vi "CVT1ParallelStaticTest.vi"() -> (3 "Unit Test Framework Results":T1)   [LabVIEW 2013, in "UnitTests.lvlib"]
uses:
  UnitTests.lvlib
  <vilib>/utf/common/utf_test_result_troll.ctl
  <vilib>/utf/common/utf_test_result.ctl
  <vilib>/utf/common/utf_test_result_failure.ctl
  <vilib>/utf/common/utf_test_comparison_operators.ctl
  <vilib>/utf/common/utf_vi_tag.ctl
  <vilib>/NI/Current Value Table/Static Write.vi
  <vilib>/NI/Current Value Table/DataTypes/I32_Static Write.vi
  <vilib>/NI/Current Value Table/Static Read.vi
  <vilib>/NI/Current Value Table/DataTypes/I32_Static Read.vi
  <vilib>/NI/Current Value Table/Type to Enum.vi
  <vilib>/NI/Current Value Table/DataTypes/I32_Type To Enum.vi
  <vilib>/NI/Current Value Table/Compatibility/TagConverter.vi
  <vilib>/NI/Current Value Table/Create Tags.vi
  <vilib>/NI/Current Value Table/FGVs/Tag Memory.vi
  <vilib>/NI/Current Value Table/Memory Block.vi
  <vilib>/NI/Current Value Table/DataTypes/I32_Memory Block.vi
  <vilib>/utf/NI_UnitTestFramework.lvlib
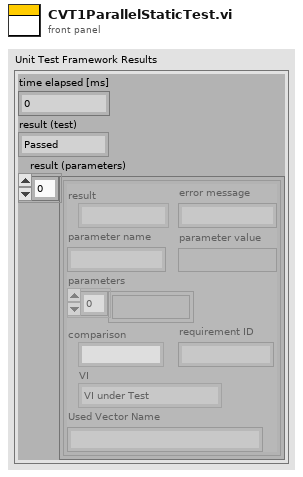
[diagram p1: front panel]
types:
  T1 = typedef "NI_UnitTestFramework.lvlib/utf_test_result_troll.ctl" = cluster{"time elapsed [ms]":u32, "result (test)":T2, "result (parameters)":T3[]}
  T2 = typedef "NI_UnitTestFramework.lvlib/utf_test_result.ctl" = enum16{"Passed", "Failed", "Error", "Skipped", "Not Processed"}
  T3 = typedef "NI_UnitTestFramework.lvlib/utf_test_result_failure.ctl" = cluster{"result":T2, "error message":string, "parameter name":string, "parameter value":variant, "parameters":variant[], "comparison":T4, "requirement ID":string, "VI":T5, "Used Vector Name":string}
  T4 = typedef "NI_UnitTestFramework.lvlib/utf_test_comparison_operators.ctl" = enum16{"=", "!=", ">", ">=", "<", "<=", "range", "symmetric tolerance", "asymmetric tolerance", "string contains", "string not contain", "array size", "string length", "array range", "by element", "array range (limit array)", "user-defined", "array contains", "array not contain", "vector length", "= (elm)", "!= (elm)", "= (case insensitive)", "!= (case insensitive)"}
  T5 = typedef "NI_UnitTestFramework.lvlib/utf_vi_tag.ctl" = enum16{"Setup VI", "VI under Test", "Teardown VI"}
  T6 = typedef "cvt_Tag Configuration.ctl" = cluster{"Name":string, "Data Type":T7, "Array":bool, "Size":u32, "Default":string, "Enum":string[], "Description":string}
  T7 = typedef "cvt_Data Types.ctl" = enum16{"Bool", "U8", "I32", "Double", "String", "Enum"}
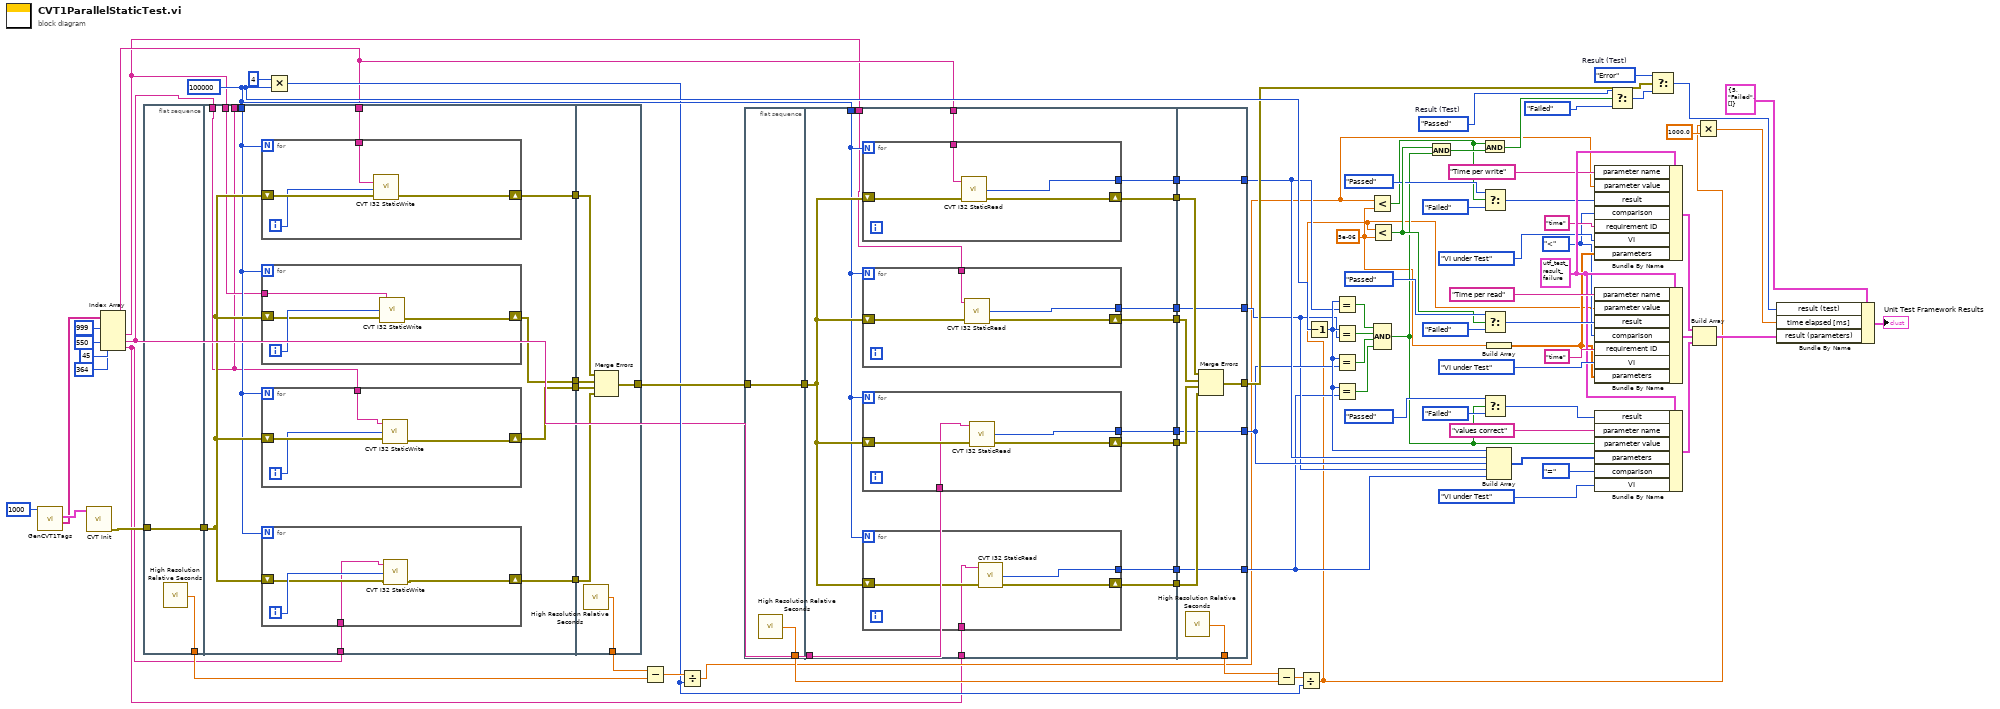
[diagram p0: block diagram]
diagram:
  w38 = T3 {"result"=enum."Passed", "error message"="", "parameter name"="", "parameter value"=variant, "parameters"=[], "comparison"=enum."=", "requirement ID"="", "VI"=enum."Setup VI", "Used Vector Name"=""} ("Unit Test Framework - result (parameters)")
  w18 = 5e-06 ("y")
  w29 = utf_test_comparison_operators."<" ("comparison")
  w70 = utf_test_result."Error"  # Result (Test)
  w13 = utf_test_result."Passed"  # Result (Test)
  w45 = 100000
  n1 = call "GenCVT1Tags.vi"("Number of Tags in"=1000) -> ("Names"=w5:string[], "Tags"=w10:T6[])  [unwired: 8 in, 1 out]
  n2 = call <vilib>:"CVT Init.vi"("Tag List"=w10) -> ("error out"=w15:errorcluster)  [unwired: 10 in]
  n3 = Index Array(array=w5, index #1=999 ("index"), index #2=550 ("index"), index #3=45 ("index"), index #4=364 ("index")) -> (element #1=w4:string, element #2=w3:string, element #3=w2:string, element #4=w1:string)
  n4 = flat-sequence {
    tunnel: [w90] -> w88
    tunnel: [w91] -> w87
    tunnel: w15 -> [w91]
    tunnel: w87 -> [w101]
    tunnel: [w100] -> w84
    tunnel: [w99] -> w83
    tunnel: [w98] -> w82
    tunnel: [w97] -> w81
    tunnel: w45 -> [w96]
    tunnel: w1 -> [w95]
    tunnel: [w93] -> _
    tunnel: w3 -> [w94]
    tunnel: w2 -> [w93]
    tunnel: w4 -> [w92]
    tunnel: [w118] -> w89
    tunnel: w84 -> [w123]
    tunnel: w83 -> [w122]
    tunnel: w82 -> [w121]
    tunnel: w81 -> [w120]
    tunnel: [w119] -> w75
    frame #0 {
      n5 = call <vilib>:"High Resolution Relative Seconds.vi"() -> ("relative seconds"=w90:dbl)
    }
    frame #1 {
      n6 = for {
        N: w96 -> [_]
        shift-right: [w117] -> w100
        shift-left: w101 -> [w116]
        tunnel: w92 -> [w114]
        i -> [w115]
        n7 = call <vilib>:"CVT I32 StaticWrite.vi"("error in (no error)"=w116, "Value"=w115, "Tag Name"=w114) -> ("error out"=w117:errorcluster)  [unwired: 2 in]
      }
      n8 = for {
        N: w96 -> [_]
        shift-right: [w103] -> w99
        shift-left: w101 -> [w104]
        tunnel: w94 -> [w102]
        i -> [w105]
        n9 = call <vilib>:"CVT I32 StaticWrite.vi"("error in (no error)"=w104, "Value"=w105, "Tag Name"=w102) -> ("error out"=w103:errorcluster)  [unwired: 2 in]
      }
      n10 = for {
        N: w96 -> [_]
        shift-right: [w113] -> w98
        shift-left: w101 -> [w112]
        tunnel: w93 -> [w110]
        i -> [w111]
        n11 = call <vilib>:"CVT I32 StaticWrite.vi"("error in (no error)"=w112, "Value"=w111, "Tag Name"=w110) -> ("error out"=w113:errorcluster)  [unwired: 2 in]
      }
      n12 = for {
        N: w96 -> [_]
        shift-right: [w107] -> w97
        shift-left: w101 -> [w108]
        tunnel: w95 -> [w106]
        i -> [w109]
        n13 = call <vilib>:"CVT I32 StaticWrite.vi"("error in (no error)"=w108, "Value"=w109, "Tag Name"=w106) -> ("error out"=w107:errorcluster)  [unwired: 2 in]
      }
    }
    frame #2 {
      n14 = call <vilib>:"High Resolution Relative Seconds.vi"() -> ("relative seconds"=w118:dbl)
      n15 = Merge Errors(w123, w122, w121, w120) -> (w119:errorcluster)
    }
  }
  n16 = Multiply(x=4, y=w45) -> (x*y=w41:i32)
  n17 = Subtract(x=w89, y=w88) -> (x-y=w43:dbl)
  n18 = Divide(x=w43, y=w41) -> (x/y=w16:dbl)
  n19 = flat-sequence {
    tunnel: [w124] -> w86
    tunnel: [w125] -> w80
    tunnel: w75 -> [w125]
    tunnel: w80 -> [w139]
    tunnel: [w138] -> w79
    tunnel: [w137] -> w78
    tunnel: [w136] -> w77
    tunnel: [w135] -> w76
    tunnel: w45 -> [w134]
    tunnel: [w133] -> w74
    tunnel: [w132] -> w52
    tunnel: [w131] -> w51
    tunnel: [w130] -> w50
    tunnel: w4 -> [w129]
    tunnel: w3 -> [w128]
    tunnel: w2 -> [w127]
    tunnel: w1 -> [w126]
    tunnel: [w165] -> w85
    tunnel: w79 -> [w159]
    tunnel: w78 -> [w158]
    tunnel: w77 -> [w157]
    tunnel: w76 -> [w156]
    tunnel: w74 -> [w163]
    tunnel: w52 -> [w161]
    tunnel: w51 -> [w162]
    tunnel: w50 -> [w164]
    tunnel: [w160] -> w40
    tunnel: [w159] -> w22
    tunnel: [w158] -> w20
    tunnel: [w157] -> w21
    tunnel: [w156] -> w19
    frame #0 {
      n20 = call <vilib>:"High Resolution Relative Seconds.vi"() -> ("relative seconds"=w124:dbl)
    }
    frame #1 {
      n21 = for {
        N: w134 -> [_]
        shift-right: [w154] -> w131
        shift-left: w139 -> [w153]
        tunnel: [w155] -> w138
        tunnel: w129 -> [w152]
        n22 = call <vilib>:"CVT I32 StaticRead.vi"("error in (no error)"=w153, "Tag Name"=w152) -> ("error out"=w154:errorcluster, "Value"=w155:i32)  [unwired: 2 in]
      }
      n23 = for {
        N: w134 -> [_]
        shift-right: [w141] -> w132
        shift-left: w139 -> [w142]
        tunnel: [w143] -> w137
        tunnel: w128 -> [w140]
        n24 = call <vilib>:"CVT I32 StaticRead.vi"("error in (no error)"=w142, "Tag Name"=w140) -> ("error out"=w141:errorcluster, "Value"=w143:i32)  [unwired: 2 in]
      }
      n25 = for {
        N: w134 -> [_]
        shift-right: [w150] -> w133
        shift-left: w139 -> [w149]
        tunnel: [w151] -> w136
        tunnel: w127 -> [w148]
        n26 = call <vilib>:"CVT I32 StaticRead.vi"("error in (no error)"=w149, "Tag Name"=w148) -> ("error out"=w150:errorcluster, "Value"=w151:i32)  [unwired: 2 in]
      }
      n27 = for {
        N: w134 -> [_]
        shift-right: [w145] -> w130
        shift-left: w139 -> [w146]
        tunnel: [w147] -> w135
        tunnel: w126 -> [w144]
        n28 = call <vilib>:"CVT I32 StaticRead.vi"("error in (no error)"=w146, "Tag Name"=w144) -> ("error out"=w145:errorcluster, "Value"=w147:i32)  [unwired: 2 in]
      }
    }
    frame #2 {
      n29 = call <vilib>:"High Resolution Relative Seconds.vi"() -> ("relative seconds"=w165:dbl)
      n30 = Merge Errors(w162, w161, w163, w164) -> (w160:errorcluster)
    }
  }
  n31 = Subtract(x=w85, y=w86) -> (x-y=w42:dbl)
  n32 = Divide(x=w42, y=w41) -> (x/y=w17:dbl)
  n33 = Decrement(x=w45) -> (x-1=w23:i32)
  n34 = Equal?(x=w23, y=w22) -> (x = y?=w46:bool)
  n35 = Equal?(x=w23, y=w20) -> (x = y?=w47:bool)
  n36 = Equal?(x=w23, y=w21) -> (x = y?=w48:bool)
  n37 = Equal?(x=w23, y=w19) -> (x = y?=w49:bool)
  n38 = Less?(x=w16, y=w18) -> (x < y?=w25:bool)
  n39 = Less?(x=w17, y=w18) -> (x < y?=w60:bool)
  n40 = Compound Arithmetic op=AND(w46, w47, w48, w49) -> (w24:bool)
  n41 = And(x=w60, y=w24) -> (x .and. y?=w34:bool)
  n42 = And(x=w25, y=w34) -> (x .and. y?=w33:bool)
  n43 = Select(t=utf_test_result."Passed" ("result"), s=w25, f=utf_test_result."Failed" ("result")) -> (s? t:f=w26:T2)
  n44 = Select(t=utf_test_result."Passed" ("result"), s=w60, f=utf_test_result."Failed" ("result")) -> (s? t:f=w63:T2)
  n45 = Select(t=utf_test_result."Passed" ("result"), s=w24, f=utf_test_result."Failed" ("result")) -> (s? t:f=w56:T2)
  n46 = Build Array(w18) -> (w30:dbl[])
  n47 = Build Array(w23, w22, w21, w20, w19) -> (w54:i32[])
  n48 = Bundle By Name(cluster=w38, "parameter name"="Time per write", "parameter value"=w16, "result"=w26, "comparison"=w29, "requirement ID"="time", "VI"=utf_vi_tag."VI under Test", "parameters"=w30) -> (w39:T3)
  n49 = Bundle By Name(cluster=w38, "parameter name"="Time per read", "parameter value"=w17, "result"=w63, "comparison"=w29, "requirement ID"="time", "VI"=utf_vi_tag."VI under Test", "parameters"=w30) -> (w37:T3)
  n50 = Bundle By Name(cluster=w38, "result"=w56, "parameter name"="values correct", "parameter value"=w24, "parameters"=w54, "comparison"=utf_test_comparison_operators."=", "VI"=utf_vi_tag."VI under Test") -> (w36:T3)
  n51 = Select(t=w13, s=w33, f=utf_test_result."Failed") -> (s? t:f=w12:T2)
  n52 = Select(t=w70, s=w40, f=w12) -> (s? t:f=w11:T2)
  n53 = Build Array(w39, w37, w36) -> (w69:T3[])
  n54 = Multiply(x=w17, y=1000.0) -> (x*y=w67:dbl)
  n55 = Bundle By Name(cluster=T1 {"time elapsed [ms]"=5, "result (test)"=enum."Failed", "result (parameters)"=[]} ("Unit Test Framework - Result"), "result (test)"=w11, "time elapsed [ms]"=w67, "result (parameters)"=w69) -> (→"Unit Test Framework Results":T1)
